vi "QI_AbortFrame.vi"(7 "path to dll":path, 8 "error in (no error)":errorcluster, 11 "Camera Handle":u32) -> (0 "error out":errorcluster, 3 "Camera Handle":u32)   [LabVIEW 2014]
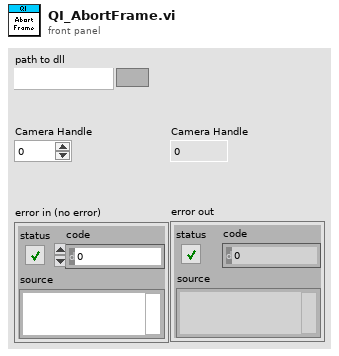
[diagram p1: front panel]
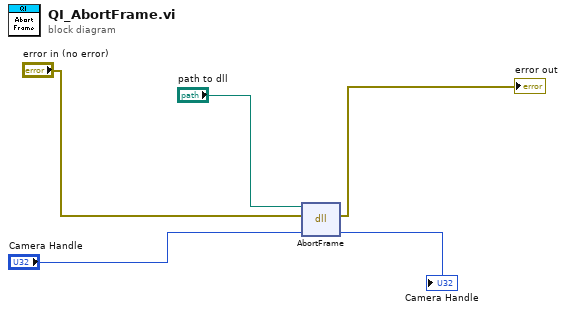
[diagram p0: block diagram]
diagram:
  n1 = dll-call lib="C:/Users/appli/Documents/Aline/octo-labview/QImaging/Release/QImaging.dll" fn="AbortFrame"(path in="path to dll", error in="error in (no error)", "handle"="Camera Handle") -> (error out=→"error out":errorcluster, "handle"=→"Camera Handle":u32)  [unwired: 2 in, 1 out]
